vi "CMI Sync V3 Error Check.vi"(8 "error in":errorcluster, 11 "VISA in":refnum<visa-resource-name>) -> (0 "error out":errorcluster, 2 "error string":string, 3 "VISA out":refnum<visa-resource-name>)   [LabVIEW 2020, in "AWG.lvlib" / "CMI Sync Unit V3.lvlib"]
doc: "Check if there is an error in the sync unit error buffer."
uses:
  CMI Sync Unit V3.lvlib
  <vilib>/Utility/error.llb/Error Cluster From Error Code.vi
  <vilib>/ErrorRing/Error Ring.xnode
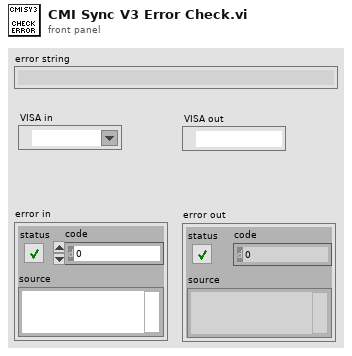
[diagram p1: front panel]
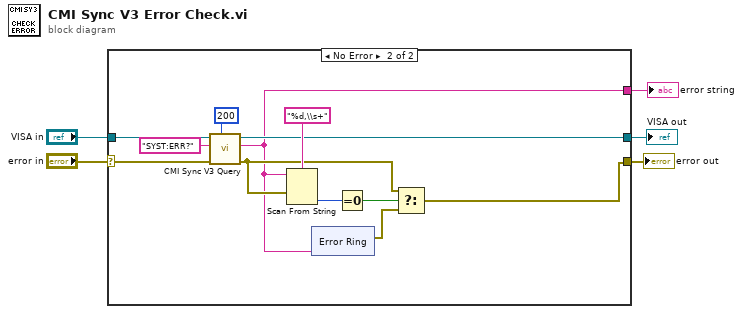
[diagram p0: block diagram]
diagram:
  n1 = case shown="No Error" "error in" {
    selector: "error in" -> [w7 w19]
    tunnel: "VISA in" -> [w6 w18]
    tunnel: [w6 w9] -> w4
    tunnel: [w7 w10] -> w2
    tunnel: [_ w8] -> w1
    frame Error {
    }
    frame No Error {
      n2 = call "CMI Sync V3 Query.vi"("read byte count (100)"=u32 200, "error in"=w19, "command"="SYST:ERR?", "VISA in"=w18) -> ("error out"=w12:errorcluster, "read buffer"=w8:string, "VISA resource name out"=w9:refnum<visa-resource-name>)  [unwired: 5 in]
      n3 = Scan From String(format string="%d,\\s+", input string=w8, error in=w12) -> (output 1=w14:i32)  [unwired: 2 in, 3 out]
      n4 = xnode "Error Ring"("parameter 0"=w8) -> ("error out"=w11:errorcluster)
      n5 = Equal To 0?(x=w14) -> (x = 0?=w13:bool)
      n6 = Select(t=w12, s=w13, f=w11) -> (s? t:f=w10:errorcluster)
    }
  }
  "error out" <- w2
  "VISA out" <- w4
  "error string" <- w1
